vi "IdentificacionObjetos3D.vi"() -> ()   [LabVIEW 2020]
doc: "En VI contiene la interfaz principal para el reconocimiento 3D de objetos. Este VI, abre la cámara seleccionada y recupera la imagen mostrandosela al usuario en tiempo real. Al presionar el botón de escanear, se manda a llamar al subVI de EscanearObjeto.vi que analiza el objeto y guarda su información en una base de datos en MySQL. El botón de identificar, manda a llamar al subVI IdentificarObjeto.vi que identifica al objeto presente en la cámara y en el recuadro de texto \"Objeto Identificado\" muestra el nombre del objeto identificado. Asimismo, el botón de Siguiente te permite moverte a otra pestaña, la cual muestra el nombre de todos los objetos guardados en la base de datos hasta el momento. En esta segunda página, se puede ingresar el nombre de un objeto que se desee de la base de datos. Esta acción se produce al presionar el botón de eliminar, siempre y cuando el texto ingresado sea válido y el objeto exista en la base."
uses:
  Estados_Maquina_Enum.ctl
  <vilib>/userdefined/High Color/IMAQdx.ctl
  <vilib>/vision/driver/NI_Vision_Acquisition_Software.lvlib
panel:
  out "Objeto Identificado 3":string caption="Objeto Identificado"
  in  "Ventanas":enum32{"Page 1", "Page 2"}(tab)
  in  "Siguiente":bool
  in  "Stop":bool
  in  "Identificar":bool
  in  "Escanear":bool
  in  "Borrar objeto":bool
  in  "Eliminar objeto":string
  in  "Anterior":bool
  out "Objetos Escaneados":string[](array[string])
  in  "Stop 2":bool caption="Stop"
  out "Imagen":T1(plugin-control)
  # "Reconocimiento de Objetos 3D"
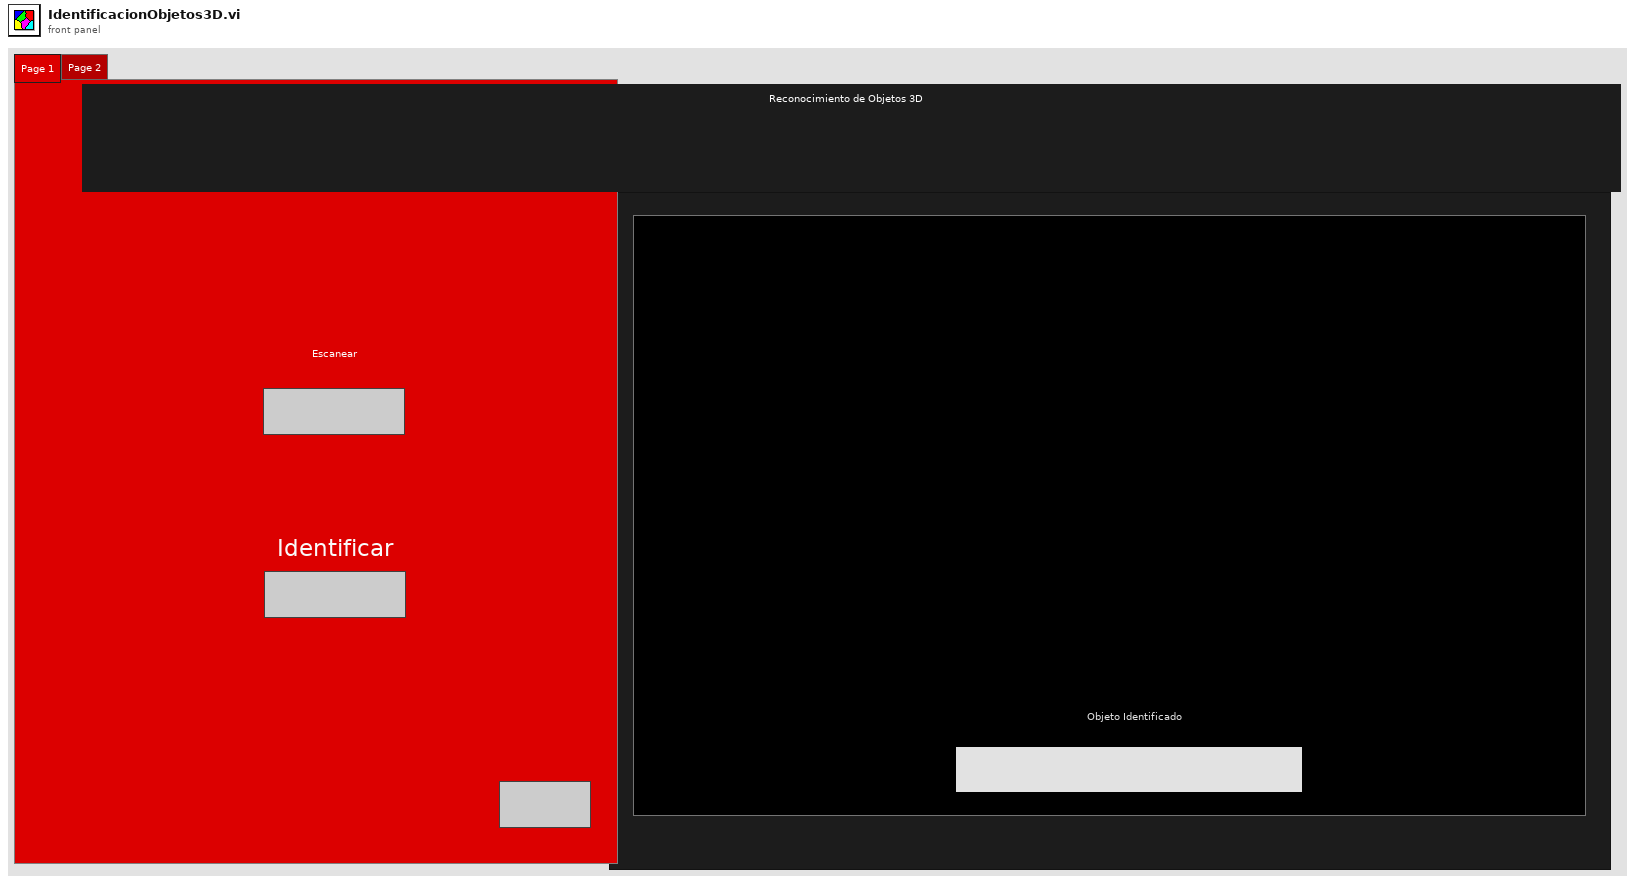
[diagram p1: front panel]
types:
  T1 = typedef "IMAQ Image.ctl" = refnum<image>
  T2 = typedef "Image Type" = u32
  T3 = typedef "IMAQdx.ctl" = refnum<k21>
  T4 = typedef "Estados_Maquina_Enum.ctl" = enum16{"Pag Anterior", "Pag Siguiente", "Actualizar lista", "Borrar Objeto", "Identificar", "Escanear", "Estado base"}
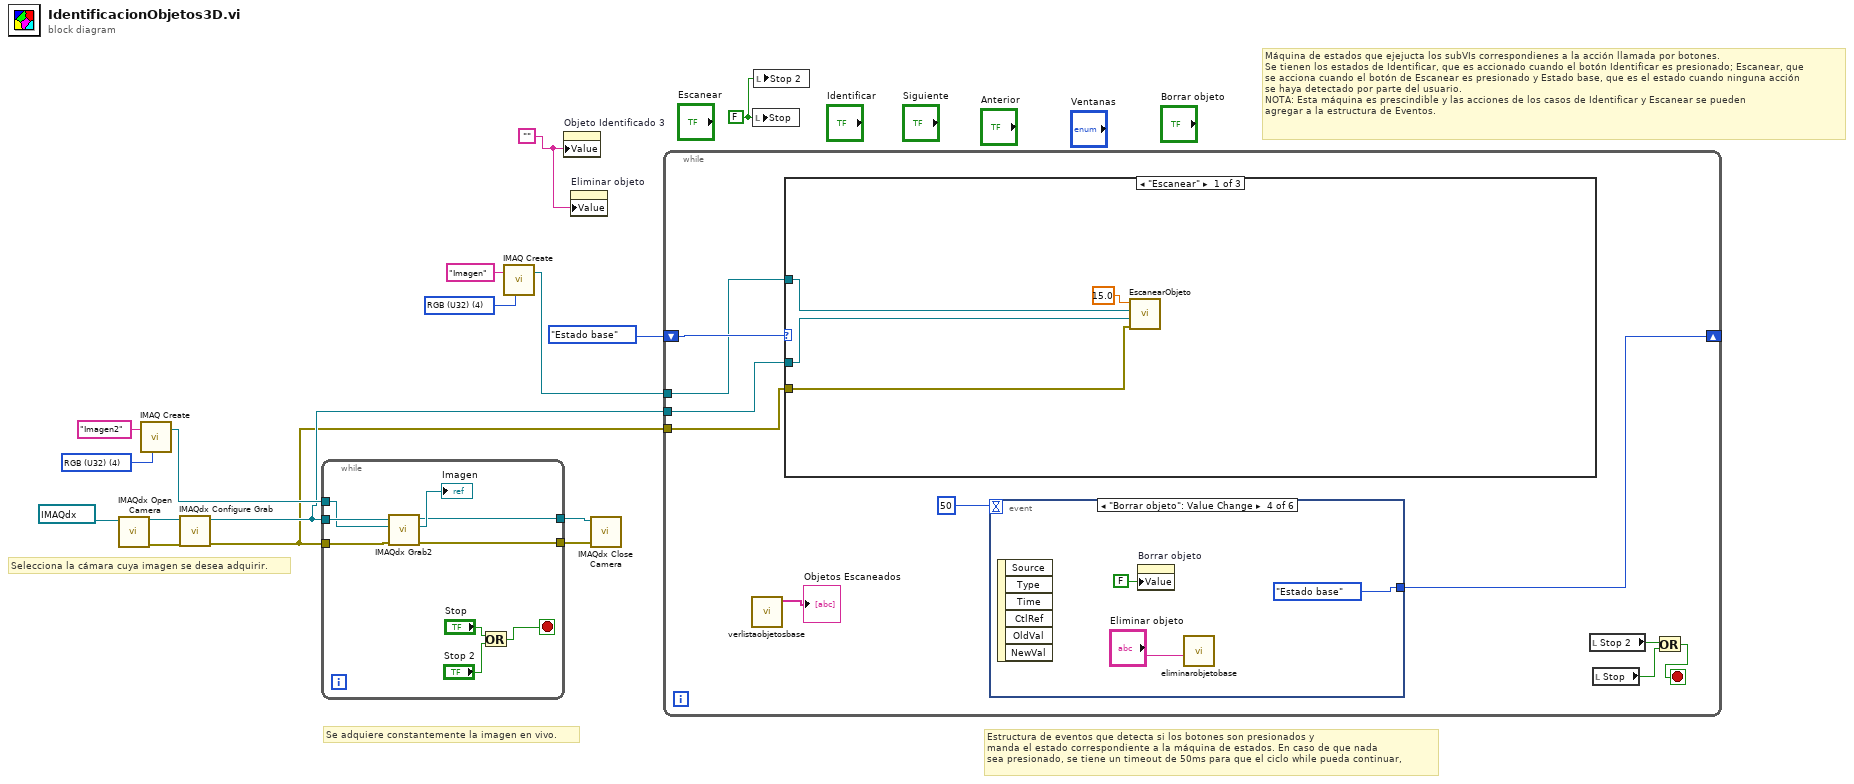
[diagram p0: block diagram]
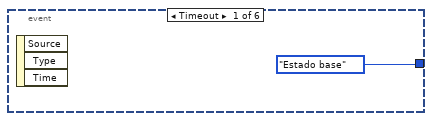
[diagram p2: hidden frame]
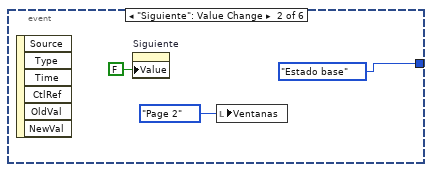
[diagram p3: hidden frame]
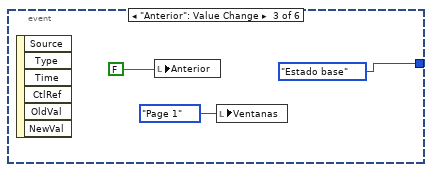
[diagram p4: hidden frame]
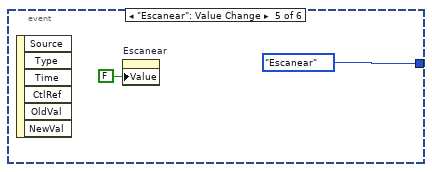
[diagram p5: hidden frame]
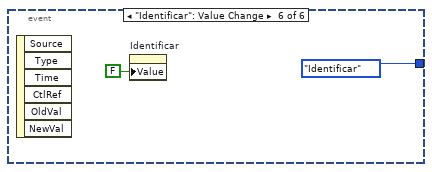
[diagram p6: hidden frame]
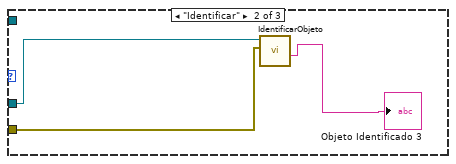
[diagram p7: hidden frame]
diagram:
  w1 = ""
  w2 = FALSE ("Stop")
  w4 = T2 4 items=["Grayscale (U8)", "Grayscale (I16)", "Grayscale (SGL)", "Complex (CSG)", "RGB (U32)", "HSL (U32)", "RGB (U64)", "Grayscale (U16)"] ("Image Type")
  w15 = T2 4 items=["Grayscale (U8)", "Grayscale (I16)", "Grayscale (SGL)", "Complex (CSG)", "RGB (U32)", "HSL (U32)", "RGB (U64)", "Grayscale (U16)"] ("Image Type")
  # "Máquina de estados que ejejucta los subVIs correspondienes a la acción llamada por botones. \nSe tienen los estados de Identificar, que es accionado cuando el botón Identificar es presionado; Escanear, que\nse acciona cuando el botón de Escanear es presionado y Estado base, que es el estado cuando ninguna acción\nse haya detectado por parte del usuario. \nNOTA: Esta máquina es prescindible y las acciones de los casos de Identificar y Escanear se pueden  \nagregar a la estructura de Eventos."
  # "Estructura de eventos que detecta si los botones son presionados y \nmanda el estado correspondiente a la máquina de estados. En caso de que nada \nsea presionado, se tiene un timeout de 50ms para que el ciclo while pueda continuar,"
  # "Selecciona la cámara cuya imagen se desea adquirir."
  # "Se adquiere constantemente la imagen en vivo."
  n1 = call <vilib>:"IMAQdx Open Camera.vi"("Session In"=T3 "cam0") -> ("error out"=w13:errorcluster, "Session Out"=w12:T3)  [unwired: 9 in]
  n2 = call "IMAQ Create"("Image Name"="Imagen2", "Image Type"=w15) -> ("New Image"=w8:T1)  [unwired: 3 in, 1 out]
  n3 = call <vilib>:"IMAQdx Configure Grab.vi"("error in"=w13, "Session In"=w12) -> ("error out"=w6:errorcluster, "Session Out"=w7:T3)  [unwired: 8 in]
  n4 = while {
    tunnel: w7 -> [w24]
    tunnel: w6 -> [w23]
    tunnel: [w22] -> w10
    tunnel: [w21] -> w9
    tunnel: w8 -> [w20]
    stop <- w17 stop-if-true
    n5 = call <vilib>:"IMAQdx Grab2.vi"("error in"=w23, "Image In"=w20, "Session In"=w24) -> ("error out"=w21:errorcluster, "Image Out"=→"Imagen":T1, "Session Out"=w22:T3)  [unwired: 5 in, 1 out]
    n6 = Or(x="Stop", y="Stop 2") -> (x .or. y?=w17:bool)
  }
  n7 = call "IMAQ Create"("Image Name"="Imagen", "Image Type"=w4) -> ("New Image"=w3:T1)  [unwired: 3 in, 1 out]
  n8 = property on="Objeto Identificado 3" class="Str"("Value"=w1) -> ()  [unwired: 2 in, 2 out]
  n9 = property on="Eliminar objeto" class="Str"("Value"=w1) -> ()  [unwired: 2 in, 2 out]
  n10 = call <vilib>:"IMAQdx Close Camera.vi"("error in"=w9, "Session In"=w10) -> ()  [unwired: 9 in, 1 out]
  n11 = while {
    shift-right: [w33] -> _
    shift-left: Estados_Maquina_Enum."Estado base" -> [w35]
    tunnel: w3 -> [w32]
    tunnel: w7 -> [w31]
    tunnel: w6 -> [w30]
    stop <- w26 stop-if-true
    n12 = call "verlistaobjetosbase.vi"() -> ("lista_objetos"=→"Objetos Escaneados":string[])  [unwired: 11 in]
    n13 = case shown="\"Escanear\"" w35 {
      tunnel: w32 -> [w51 _ _]
      tunnel: w31 -> [w52 w56 _]
      tunnel: w30 -> [w50 w55 _]
      frame "Escanear" {
        n14 = call "EscanearObjeto.vi"("Error in"=w50, "Sesion"=w52, "Imagen"=w51, "Ángulo por foto:"=15.0) -> ()  [unwired: 4 in, 4 out]
      }
      frame "Identificar" {
        n15 = call "IdentificarObjeto.vi"("Error in"=w55, "Session In"=w56) -> ("Objeto Detectado"=→"Objeto Identificado 3":string)  [unwired: 8 in, 1 out]
      }
      frame "Estado base", Default {
      }
    }
    n16 = event shown="[3] \"Borrar objeto\": Value Change" {
      selector: _ -> [_ _ _ _ _ _]
      dyn-events: _ -> [_ _ _ _ _ _]
      timeout: 50 -> [_ _ _ _ _ _]
      tunnel: [Estados_Maquina_Enum."Estado base" Estados_Maquina_Enum."Estado base" Estados_Maquina_Enum."Estado base" Estados_Maquina_Enum."Estado base" Estados_Maquina_Enum."Escanear" Estados_Maquina_Enum."Identificar"] -> w33
      event Timeout {
        n17 = event-data() -> ()  [unwired: 1 in, 3 out]
      }
      event "Siguiente": Value Change {
        n18 = event-data() -> ()  [unwired: 1 in, 6 out]
        n19 = property on="Siguiente" class="Bool (strict)"("Value"=FALSE ("Mover a Der")) -> ()  [unwired: 2 in, 2 out]
        n20 = local write "Ventanas"(enum32{"Page 1", "Page 2"}."Page 2" ("Tab Control")) -> ()
      }
      event "Anterior": Value Change {
        n21 = event-data() -> ()  [unwired: 1 in, 6 out]
        n22 = local write "Anterior"(FALSE ("Mover a Der")) -> ()
        n23 = local write "Ventanas"(enum32{"Page 1", "Page 2"}."Page 1" ("Tab Control")) -> ()
      }
      event "Borrar objeto": Value Change {
        n24 = event-data() -> ()  [unwired: 1 in, 6 out]
        n25 = property on="Borrar objeto" class="Bool (strict)"("Value"=FALSE ("Borrar objeto")) -> ()  [unwired: 2 in, 2 out]
        n26 = call "eliminarobjetobase.vi"("Nombre objeto a eliminar"="Eliminar objeto") -> ()  [unwired: 11 in]
      }
      event "Escanear": Value Change {
        n27 = event-data() -> ()  [unwired: 1 in, 6 out]
        n28 = property on="Escanear" class="Bool (strict)"("Value"=FALSE ("Escanear")) -> ()  [unwired: 2 in, 2 out]
      }
      event "Identificar": Value Change {
        n29 = event-data() -> ()  [unwired: 1 in, 6 out]
        n30 = property on="Identificar" class="Bool (strict)"("Value"=FALSE ("Identificar")) -> ()  [unwired: 2 in, 2 out]
      }
    }
    n31 = local read "Stop 2"() -> (w28:bool)
    n32 = local read "Stop"() -> (w27:bool)
    n33 = Or(x=w28, y=w27) -> (x .or. y?=w26:bool)
  }
  n34 = local write "Stop"(w2) -> ()
  n35 = local write "Stop 2"(w2) -> ()
